vi "Select Mode Est Settings.vi"(10 "notifier":refnum<notifier>) -> (2 "Mode Estimator Processing Settings out":T1={"Low-Pass Filter Order"=5, "Downsampling Ratio"=10.0, "LPF Cut-off Frequency [Hz]"=2.5, "Sampling Frequency (Hz)"=50.0, "Parcel Length (Simulation)"=30000, "Detrend Cut-off Frequency (Hz)"=0.05, "AR Order"=25, "MA Order "=10, "Lower Frequency [Hz]"=0.08, "Upper Frequency [Hz]"=2.0, "Upper Damping [%]"=20.0, "Lower Damping [%]"=0.0, "Std Threshold"=1.35, "Length of Spectra [s]"=12.0, "Refresh Rate [s]"=0, "Number of critical modes"=1})   [LabVIEW 2017]
uses:
  Mode Est Processing Settings.ctl
panel:
  in  "Mode Estimation Settings":T1={"Low-Pass Filter Order"=5, "Downsampling Ratio"=10.0, "LPF Cut-off Frequency [Hz]"=2.5, "Sampling Frequency (Hz)"=50.0, "Parcel Length (Simulation)"=30000, "Detrend Cut-off Frequency (Hz)"=0.05, "AR Order"=25, "MA Order "=10, "Lower Frequency [Hz]"=0.08, "Upper Frequency [Hz]"=2.0, "Upper Damping [%]"=20.0, "Lower Damping [%]"=0.0, "Std Threshold"=1.35, "Length of Spectra [s]"=12.0, "Refresh Rate [s]"=0, "Number of critical modes"=1}
  in  "OK Button":bool
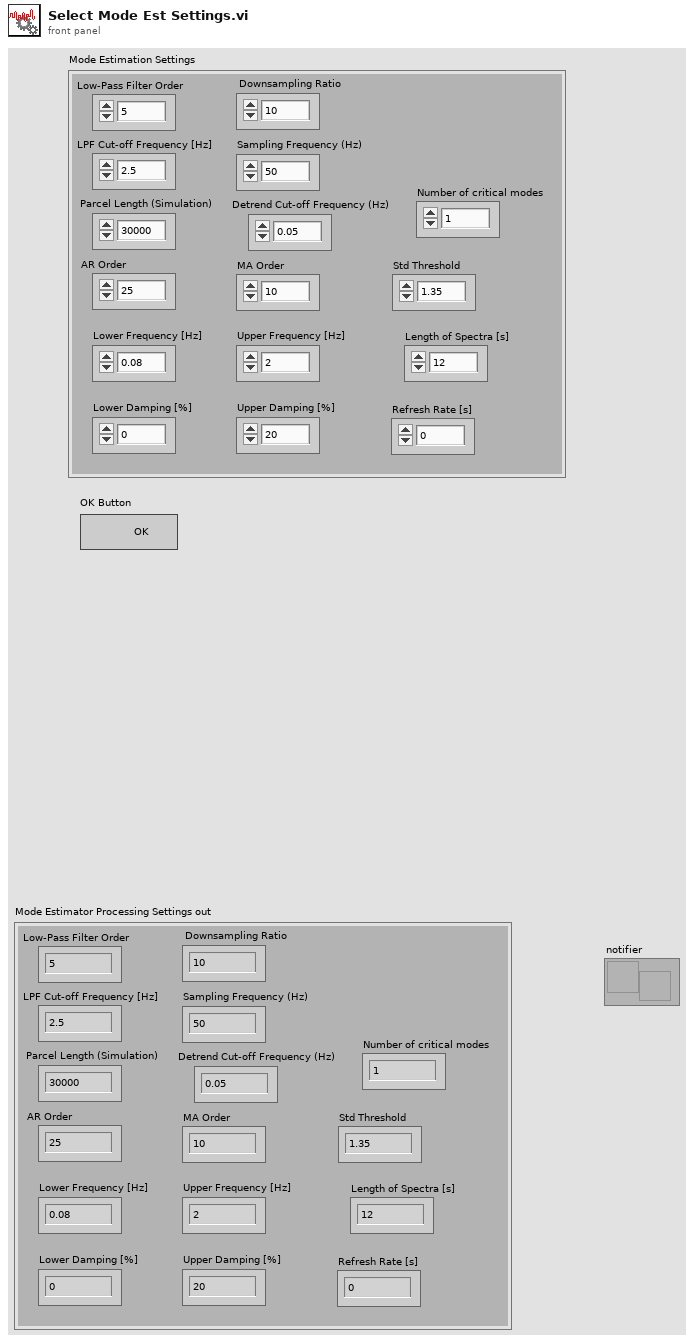
[diagram p1: front panel]
types:
  T1 = typedef "Mode Est Processing Settings.ctl" = cluster{"Low-Pass Filter Order":i32, "Downsampling Ratio":dbl, "LPF Cut-off Frequency [Hz]":dbl, "Sampling Frequency (Hz)":dbl, "Parcel Length (Simulation)":i32, "Detrend Cut-off Frequency (Hz)":dbl, "AR Order":i32, "MA Order ":i32, "Lower Frequency [Hz]":dbl, "Upper Frequency [Hz]":dbl, "Upper Damping [%]":dbl, "Lower Damping [%]":dbl, "Std Threshold":dbl, "Length of Spectra [s]":dbl, "Refresh Rate [s]":i32, "Number of critical modes":i32}
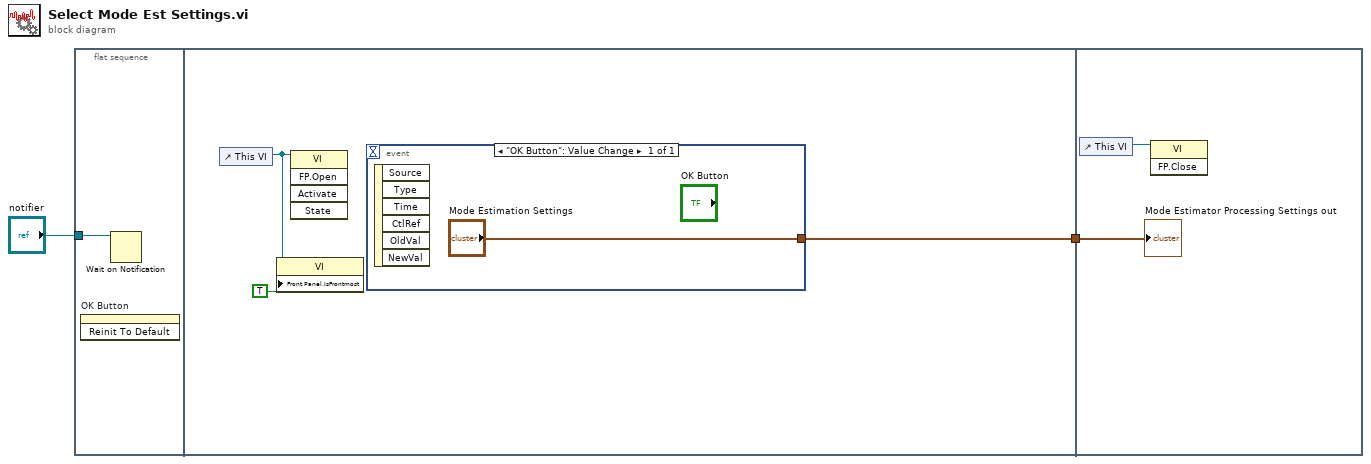
[diagram p0: block diagram]
diagram:
  n1 = flat-sequence {
    tunnel: "notifier" -> [w3]
    tunnel: [w4] -> w1
    tunnel: w1 -> [w8]
    frame #0 {
      n2 = invoke on="OK Button" class="Bool" method="Reinit To Default"() -> ()  [unwired: 3 in, 3 out]
      n3 = Wait on Notification(notifier=w3) -> ()  [unwired: 3 in, 4 out]
    }
    frame #1 {
      n4 = control-ref of="This VI"() -> (w6:refnum<vi>)
      n5 = property class="VI"(reference=w6, "Front Panel.IsFrontmost"=TRUE ("Front Panel Window:Is Frontmost")) -> ()  [unwired: 1 in, 2 out]
      n6 = invoke class="VI" method="FP.Open"(reference=w6) -> ()  [unwired: 4 in, 5 out]
      n7 = event shown="[0] \"OK Button\": Value Change" {
        selector: _ -> [_]
        dyn-events: _ -> [_]
        timeout: _ -> [_]
        tunnel: ["Mode Estimation Settings"] -> w4
        event "OK Button": Value Change {
          n8 = event-data() -> ()  [unwired: 1 in, 6 out]
        }
      }
    }
    frame #2 {
      n9 = control-ref of="This VI"() -> (w9:refnum<vi>)
      n10 = invoke class="VI" method="FP.Close"(reference=w9) -> ()  [unwired: 2 in, 3 out]
      "Mode Estimator Processing Settings out" <- w8
    }
  }
